vi "XGB 연속 쓰기(BCC).vi"() -> ()   [LabVIEW 2014]
uses:
  <vilib>/Instr/_visa.llb/VISA Configure Serial Port (Instr).vi
panel:
  in  "VISA resource name":refnum<visa-resource-name>="COM13"
  out "error out":errorcluster={"status"=FALSE, "code"=1073676294, "source"="XGB 읽기.vi 안에 VISA 읽기"} caption="에러 출력"
  out "응답 프레임":string="\u000600RSB016430313233323330303233303032333030323330303233303000000000000000000000000000000000000000000000000000000000000000000000000000000000000000000000000000000000000000000000000000000000000000000000000000000000\u0003"
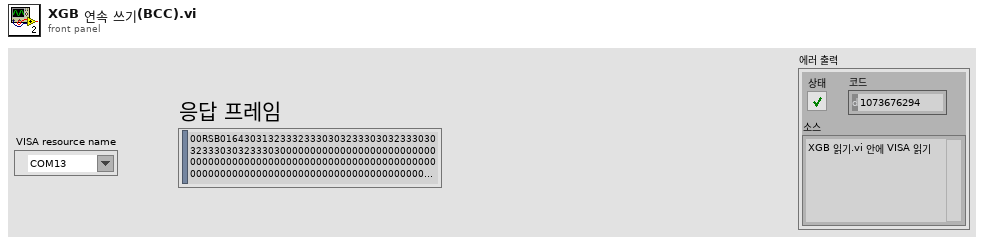
[diagram p1: front panel]
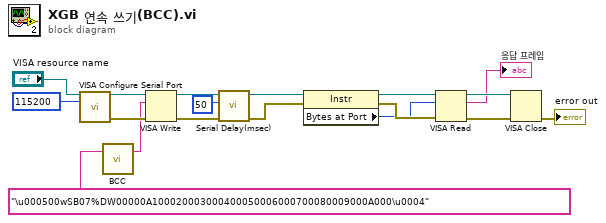
[diagram p0: block diagram]
diagram:
  n1 = call-poly "VISA Configure Serial Port"("VISA resource name"="VISA resource name", "baud rate (9600)"=u32 115200 ("baud rate")) -> ("VISA resource name out"=w9:refnum<visa-resource-name>, "error out"=w8:errorcluster)  [unwired: 12 in]
  n2 = call "BCC.vi"("Message"="\u000500wSB07%DW00000A100020003000400050006000700080009000A000\u0004" ("요구 프레임")) -> ("Message with BCC"=w1:string)  [unwired: 1 in, 1 out]
  n3 = VISA Write(VISA resource name=w9, write buffer=w1, error in (no error)=w8) -> (VISA resource name out=w16:refnum<visa-resource-name>, error out=w13:errorcluster)  [unwired: 1 out]
  n4 = call "Serial Delay(msec).vi"("에러 입력(에러 없음)"=w13, "milliseconds to wait"=u32 50, "VISA 참조 번호 입력"=w16) -> ("에러 출력"=w14:errorcluster, "VISA 참조 번호 출력"=w15:refnum<visa-resource-name>)  [unwired: 7 in]
  n5 = property class="Instr"(reference=w15, error in=w14) -> (reference out=w17:refnum<visa-resource-name>, error out=w18:errorcluster, "Bytes at Port"=w3:u32)
  n6 = VISA Read(VISA resource name=w17, byte count=w3, error in (no error)=w18) -> (VISA resource name out=w7:refnum<visa-resource-name>, read buffer=→"응답 프레임":string, error out=w6:errorcluster)  [unwired: 1 out]
  n7 = VISA Close(VISA resource name=w7, error in (no error)=w6) -> (error out=→"error out":errorcluster)
